vi "DecisionTreeTests.vi"() -> ()   [LabVIEW 2020]
uses:
  controls/DecisionTree.ctl
  controls/Gameboard Data.ctl
  controls/DecisionTreeRecord.ctl
  controls/Player.ctl
panel:
  in  "Current Player":T1=enum."Player 2"
  in  "Gameboard":T2=[enum."Player 1", enum."Player 2", enum."None", enum."None", enum."Player 1", enum."None", enum."None", enum."None", enum."None"]
  out "DecisionTree Out":T3
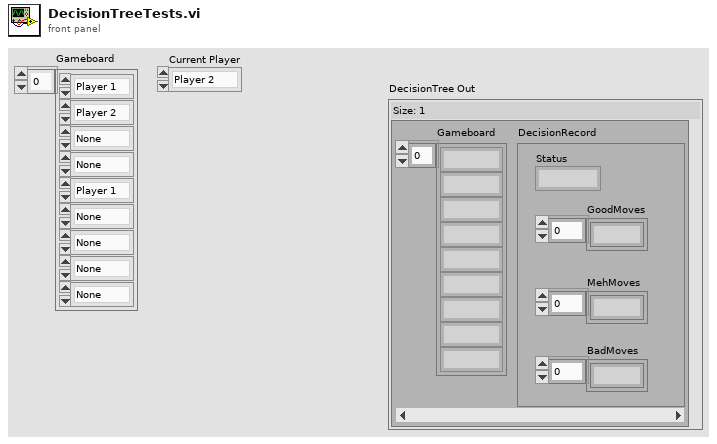
[diagram p1: front panel]
types:
  T1 = typedef "Player.ctl" = enum16{"None", "Player 1", "Player 2"}
  T2 = typedef "Gameboard Data.ctl" = enum16{"None", "Player 1", "Player 2"}[]
  T3 = typedef "DecisionTree.ctl" = map{T2, T4}
  T4 = typedef "DecisionTreeRecord.ctl" = cluster{"Status":T1, "GoodMoves":i8[], "MehMoves":i8[], "BadMoves":i8[]}
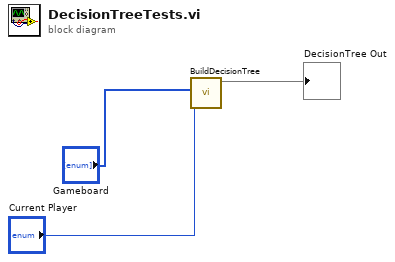
[diagram p0: block diagram]
diagram:
  n1 = call "BuildDecisionTree.vi"("Current Player"="Current Player", "Gameboard"="Gameboard") -> ("DecisionTree Out"=→"DecisionTree Out":T3)  [unwired: 7 in, 2 out]
